vi "Init_Screen_Ctls.vi"(8 "entrée d'erreur (pas d'erreur)":errorcluster, 10 "Cluster to load":refnum<vi>, 11 "VI ref":refnum<vi>) -> (0 "error out":errorcluster, 2 "UI matched items":refnum<vi>[](array[refnum]), 3 "VI ref out":refnum<vi>)   [LabVIEW 2020, in "UI_Actor.lvlib" / "UI_Actor.lvclass"]
uses:
  UI_Actor.lvclass
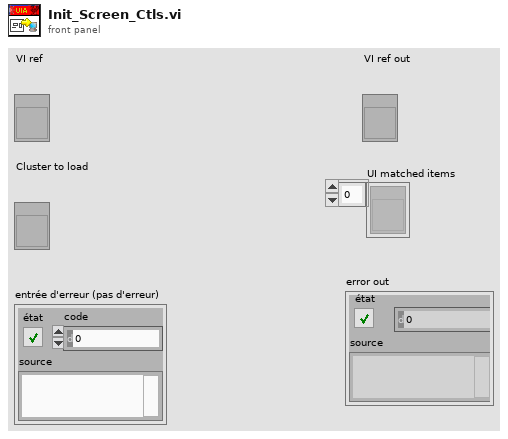
[diagram p1: front panel]
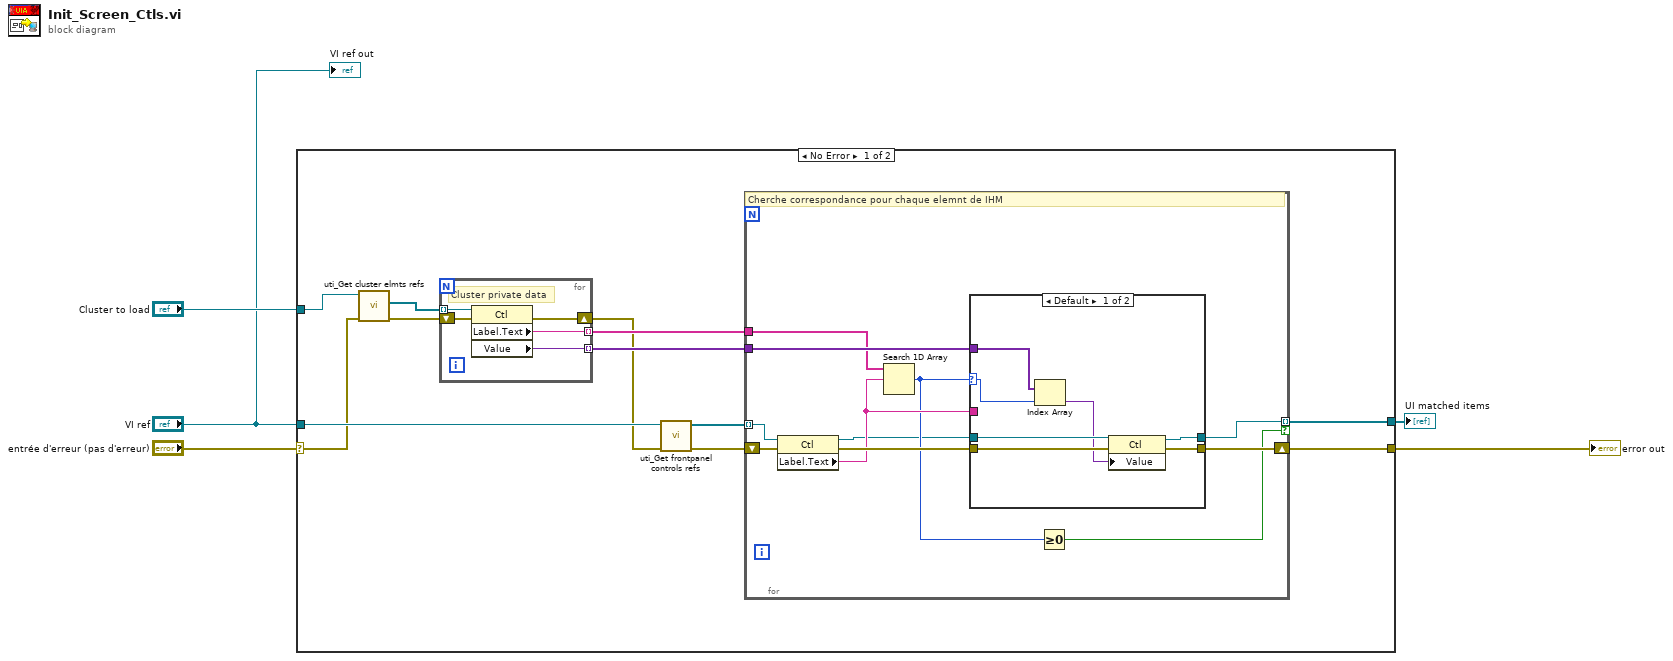
[diagram p0: block diagram]
diagram:
  n1 = case shown="No Error" "entrée d'erreur (pas d'erreur)" {
    selector: "entrée d'erreur (pas d'erreur)" -> [w7 w43]
    tunnel: "VI ref" -> [w14 _]
    tunnel: [w11 w43] -> w5
    tunnel: "Cluster to load" -> [w9 _]
    tunnel: [w10 _] -> w1
    frame No Error {
      n2 = call "uti_Get cluster elmts refs.vi"("entrée d'erreur (pas d'erreur)"=w7, "Cluster ref in"=w9) -> ("error out"=w6:errorcluster, "Controls[]"=w8:refnum<vi>[])  [unwired: 7 in, 1 out]
      n3 = for {
        tunnel: w8 -> [w22] mode=indexing
        tunnel: [w21] -> w16 mode=indexing
        tunnel: [w20] -> w17 mode=indexing
        shift-right: [w18] -> w13
        shift-left: w6 -> [w19]
        # "Cluster private data"
        n4 = property class="Ctl"(reference=w22, error in=w19) -> (error out=w18:errorcluster, "Label.Text"=w21:string, "Value"=w20:variant)  [unwired: 1 out]
      }
      n5 = call "uti_Get frontpanel controls refs.vi"("error in (no error)"=w13, "VI ref"=w14) -> ("error out"=w12:errorcluster, "Controls[]"=w15:refnum<vi>[])  [unwired: 8 in]
      n6 = for {
        tunnel: w15 -> [w30] mode=indexing
        tunnel: w16 -> [w31]
        tunnel: w17 -> [w33]
        shift-right: [w32] -> w11
        shift-left: w12 -> [w29]
        tunnel: [w23] -> w10 mode=indexing if=w25
        # "Cherche correspondance pour chaque elemnt de IHM"
        n7 = property class="Ctl"(reference=w30, error in=w29) -> (reference out=w24:refnum<vi>, error out=w28:errorcluster, "Label.Text"=w27:string)
        n8 = Search 1D Array(1D array=w31, element=w27) -> (index of element=w26:i32)  [unwired: 1 in]
        n9 = case shown="Default" w26 {
          selector: w26 -> [w35 _]
          tunnel: w33 -> [w40 _]
          tunnel: [w39 w42] -> w32
          tunnel: w24 -> [w38 w41]
          tunnel: w28 -> [w37 w42]
          tunnel: w27 -> [_ _]
          tunnel: [w34 w41] -> w23
          frame Default {
            n10 = Index Array(array=w40, index=w35) -> (element=w36:variant)
            n11 = property class="Ctl"(reference=w38, error in=w37, "Value"=w36) -> (reference out=w34:refnum<vi>, error out=w39:errorcluster)
          }
          frame -1 {
          }
        }
        n12 = Greater Or Equal To 0?(x=w26) -> (x >= 0?=w25:bool)
      }
    }
    frame Error {
    }
  }
  "error out" <- w5
  "UI matched items" <- w1
  "VI ref out" <- "VI ref"
